vi "Lectura Silicon 6 bytes.vi"() -> ()   [LabVIEW 2013]
uses:
  <vilib>/Instr/_visa.llb/VISA Configure Serial Port (Instr).vi
  <vilib>/Instr/_visa.llb/VISA Serial Break (Instr).vi
panel:
  out "array 2":string[](array[string])
  out "read buffer 2":string
  out "Waveform Graph 2":waveform(i32)(graph)
  in  "Reiniciar":bool
  out "mps":dbl
  out "Array 3":string[](array[string])
  out "Array 2":timestamp[](array[timestamp])
  out "unsigned byte array":u8[](array[numeric])
  out "x != y?":bool
  in  "Array":bool[](array[boolean])=[FALSE, FALSE, FALSE, FALSE, FALSE, FALSE, FALSE, TRUE]
  out "Waveform Graph":waveform(i32)(graph)
  out "Boolean array":bool[][](array[boolean])
  out "array":string[](array[string])
  in  "stop":bool
  out "read buffer":string
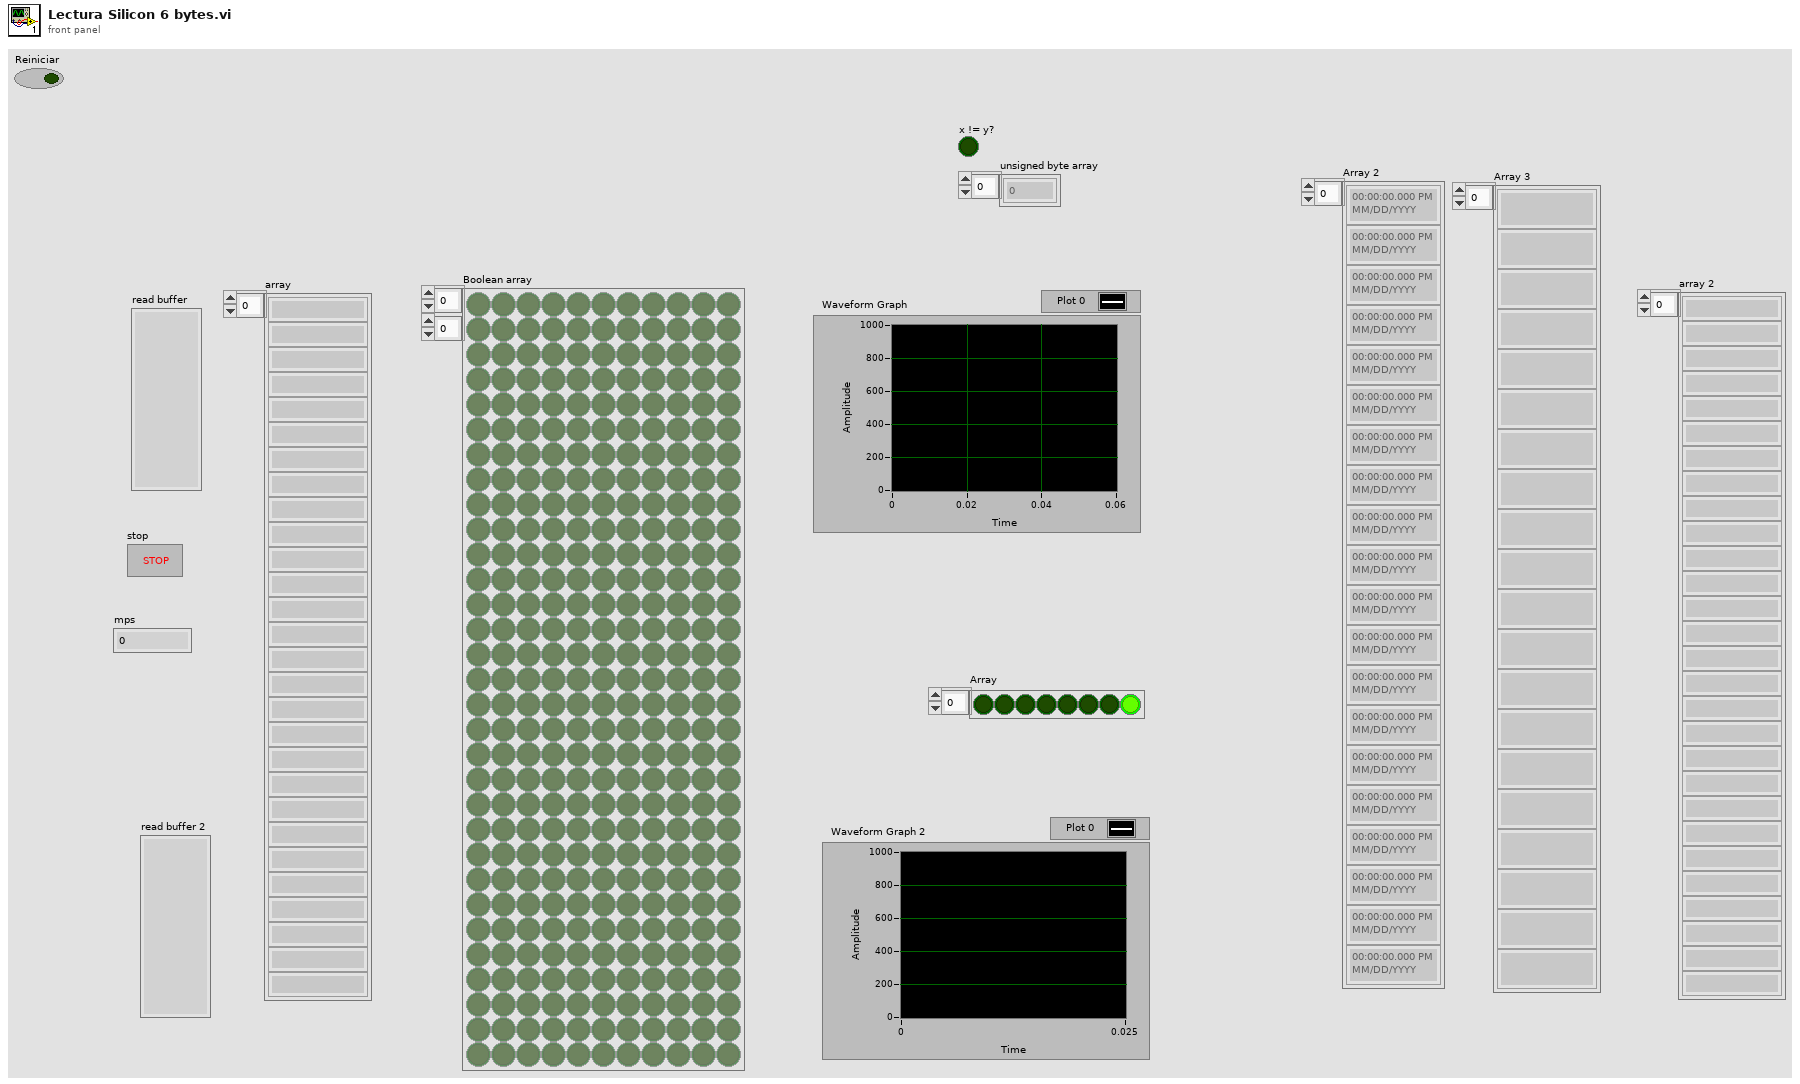
[diagram p1: front panel]
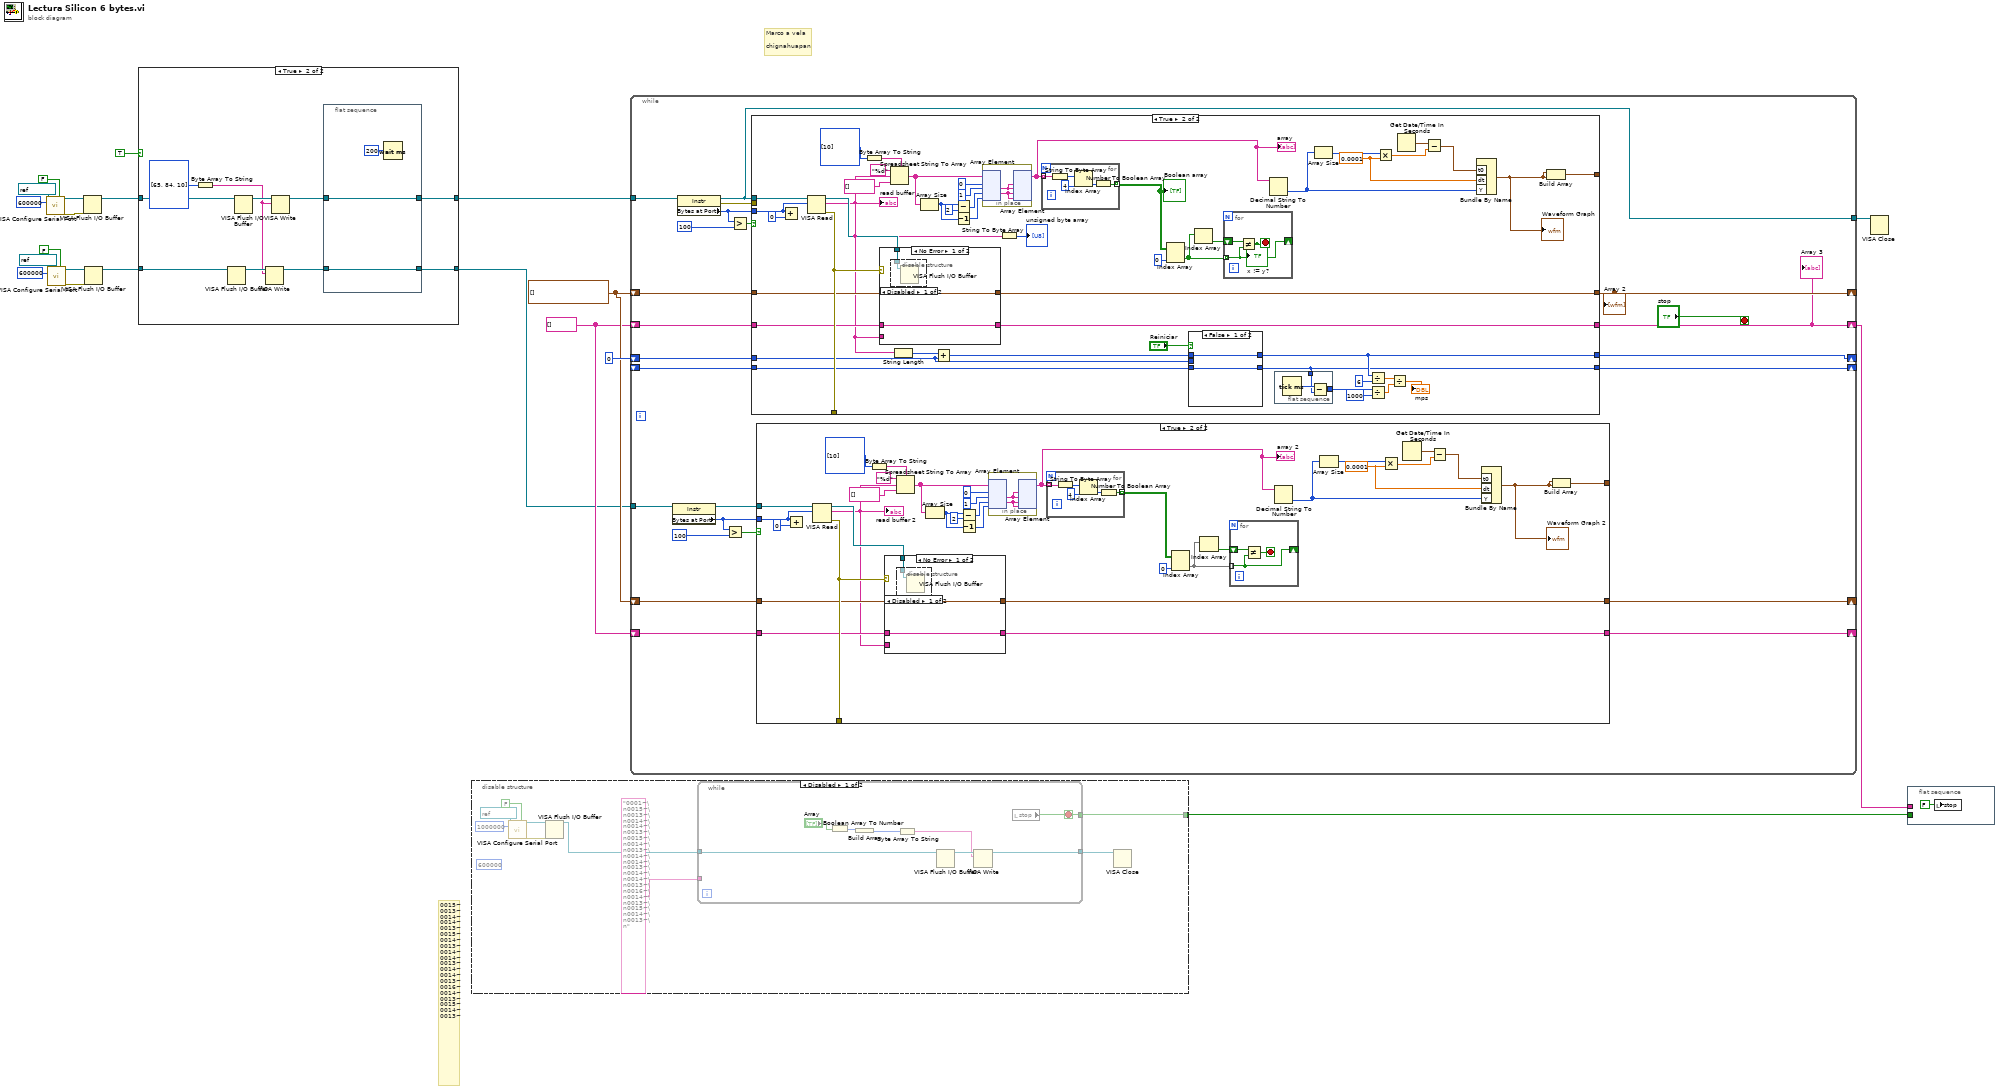
[diagram p0: block diagram]
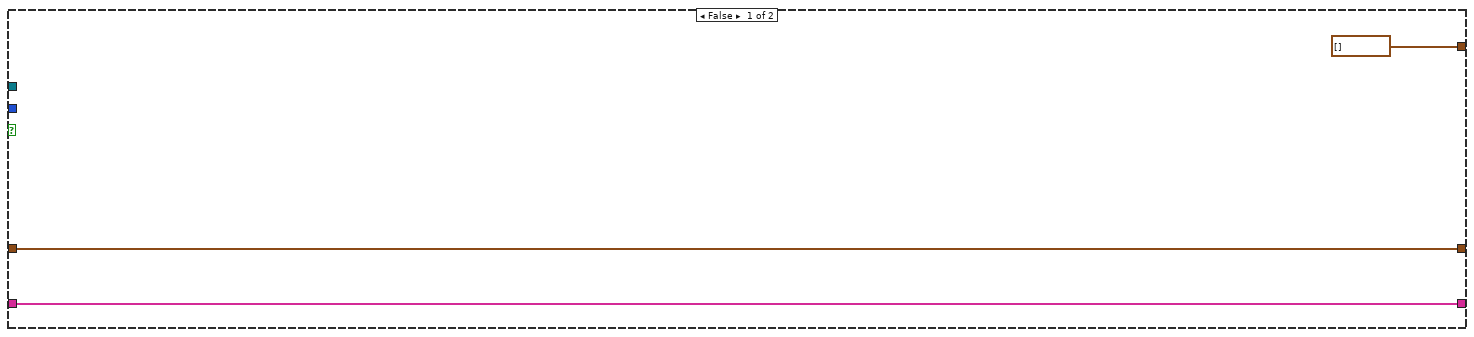
[diagram p4: hidden frame]
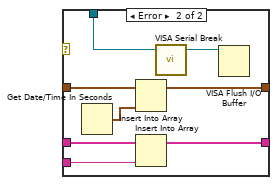
[diagram p6: hidden frame]
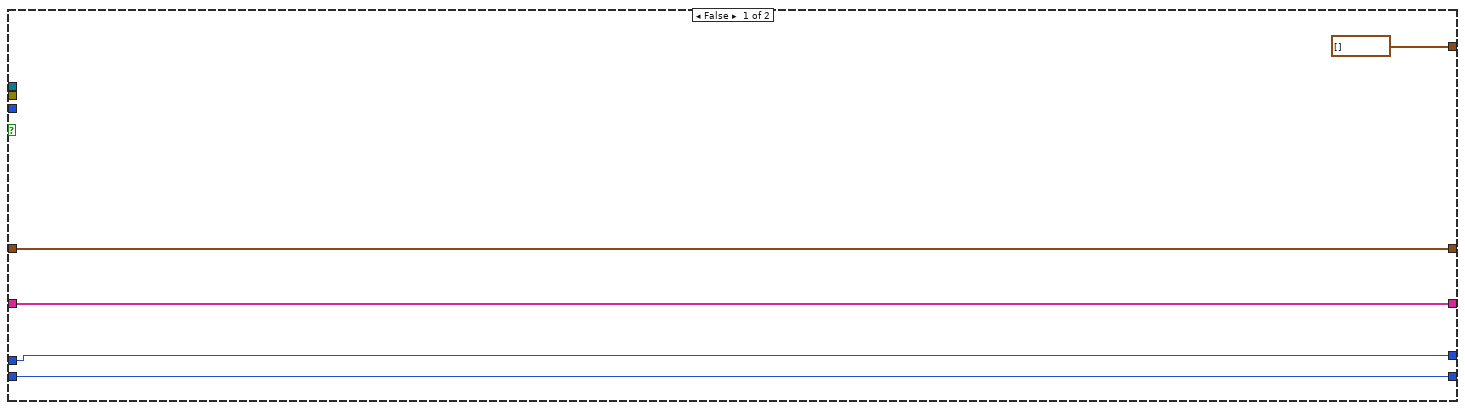
[diagram p7: hidden frame]
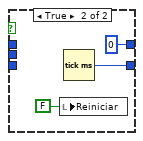
[diagram p8: hidden frame]
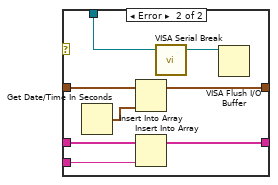
[diagram p10: hidden frame]
diagram:
  w8 = string[] []
  w9 = timestamp[] []
  # "Marco a vela\n\nchignahuapan"
  # "0015~\n0013~\n0014~\n0014~\n0013~\n0015~\n0014~\n0013~\n0014~\n0014~\n0013~\n0014~\n0014~\n0013~\n0016~\n0014~\n0013~\n0015~\n0014~\n0013~"
  n1 = call-poly "VISA Configure Serial Port"("VISA resource name"=refnum<visa-resource-name> "COM4", "Enable Termination\nChar (T)"=FALSE ("Enable Termination\nChar (T)"), "baud rate (9600)"=u32 600000) -> ("VISA resource name out"=w19:refnum<visa-resource-name>, "error out"=w18:errorcluster)  [unwired: 11 in]
  n2 = call-poly "VISA Configure Serial Port"("VISA resource name"=refnum<visa-resource-name> "COM5", "Enable Termination\nChar (T)"=FALSE ("Enable Termination\nChar (T)"), "baud rate (9600)"=u32 600000) -> ("VISA resource name out"=w5:refnum<visa-resource-name>, "error out"=w6:errorcluster)  [unwired: 11 in]
  n3 = VISA Flush I/O Buffer(VISA resource name=w19, error in (no error)=w18) -> (VISA resource name out=w12:refnum<visa-resource-name>)  [unwired: 1 in, 1 out]
  n4 = VISA Flush I/O Buffer(VISA resource name=w5, error in (no error)=w6) -> (VISA resource name out=w2:refnum<visa-resource-name>)  [unwired: 1 in, 1 out]
  n5 = case shown="True" TRUE {
    tunnel: w12 -> [w23 w32]
    tunnel: [w23 w29] -> w11
    tunnel: w2 -> [w22 w27]
    tunnel: [w22 w24] -> w1
    frame False {
    }
    frame True {
      n6 = Byte Array To String(unsigned byte array=u8[] [65, 84, 10]) -> (string=w26:string)
      n7 = VISA Flush I/O Buffer(VISA resource name=w27) -> (VISA resource name out=w28:refnum<visa-resource-name>)  [unwired: 2 in, 1 out]
      n8 = VISA Flush I/O Buffer(VISA resource name=w32) -> (VISA resource name out=w33:refnum<visa-resource-name>)  [unwired: 2 in, 1 out]
      n9 = VISA Write(VISA resource name=w28, write buffer=w26) -> (VISA resource name out=w25:refnum<visa-resource-name>)  [unwired: 1 in, 2 out]
      n10 = VISA Write(VISA resource name=w33, write buffer=w26) -> (VISA resource name out=w30:refnum<visa-resource-name>)  [unwired: 1 in, 2 out]
      n11 = flat-sequence {
        tunnel: w30 -> [w36]
        tunnel: [w36] -> w29
        tunnel: w25 -> [w34]
        tunnel: [w34] -> w24
        frame #0 {
          n12 = Wait (ms)(milliseconds to wait=u32 200) -> ()  [unwired: 1 out]
        }
      }
    }
  }
  n13 = disable-structure shown="Disabled" {
    disable-tunnel: [w40 _] -> w14
    frame Disabled {
      (unwired) u32 600000 ("baud rate (9600)")
      n14 = call-poly "VISA Configure Serial Port"("VISA resource name"=refnum<visa-resource-name> "COM5", "Enable Termination\nChar (T)"=FALSE ("Enable Termination\nChar (T)"), "baud rate (9600)"=u32 1000000) -> ("VISA resource name out"=w43:refnum<visa-resource-name>, "error out"=w44:errorcluster)  [unwired: 11 in]
      n15 = VISA Flush I/O Buffer(VISA resource name=w43, error in (no error)=w44) -> (VISA resource name out=w41:refnum<visa-resource-name>)  [unwired: 1 in, 1 out]
      n16 = while {
        tunnel: w41 -> [w49]
        tunnel: [w48] -> w40
        tunnel: "0001~\n0015~\n0013~\n0014~\n0014~\n0013~\n0015~\n0014~\n0013~\n0014~\n0014~\n0013~\n0014~\n0014~\n0013~\n0016~\n0014~\n0013~\n0015~\n0014~\n0013~\n" ("read buffer") -> [_]
        tunnel: [w47] -> w38
        stop <- w48 stop-if-true
        n17 = Boolean Array To Number(Boolean array="Array") -> (number=w52:u8)
        n18 = Build Array(w52) -> (w53:u8[])
        n19 = Byte Array To String(unsigned byte array=w53) -> (string=w46:string)
        n20 = VISA Flush I/O Buffer(VISA resource name=w49) -> (VISA resource name out=w50:refnum<visa-resource-name>)  [unwired: 2 in, 1 out]
        n21 = VISA Write(VISA resource name=w50, write buffer=w46) -> (VISA resource name out=w47:refnum<visa-resource-name>)  [unwired: 1 in, 2 out]
        n22 = local read "stop"() -> (w48:bool)
      }
      n23 = VISA Close(VISA resource name=w38) -> ()  [unwired: 1 in, 1 out]
    }
    frame Enabled {
    }
  }
  n24 = while {
    tunnel: w11 -> [w73]
    tunnel: [w72] -> w16
    shift-right: [w70] -> _
    shift-left: w9 -> [w71]
    shift-right: [w68] -> w15
    shift-left: w8 -> [w69]
    shift-right: [w65] -> _
    shift-left: u32 0 ("length") -> [w66]
    shift-right: [w64] -> _
    shift-left: _ -> [w63]
    shift-right: [w60] -> _
    shift-left: w9 -> [w62]
    shift-right: [w59] -> _
    shift-left: w8 -> [w61]
    tunnel: w1 -> [w56]
    stop <- "stop" stop-if-true
    n25 = property class="Instr"(reference=w56) -> (reference out=w55:refnum<visa-resource-name>, "Bytes at Port"=w54:u32)  [unwired: 1 in, 1 out]
    n26 = property class="Instr"(reference=w73) -> (reference out=w72:refnum<visa-resource-name>, error out=w76:errorcluster, "Bytes at Port"=w77:u32)  [unwired: 1 in]
    n27 = Greater?(x=w54, y=u32 100) -> (0:w57:bool)
    n28 = Greater?(x=w77, y=u32 100) -> (0:w67:bool)
    n29 = case shown="True" w67 {
      tunnel: w72 -> [_ w164]
      tunnel: w77 -> [_ w156]
      tunnel: [waveform(dbl)[] [] w180] -> _
      tunnel: w76 -> [_ _]
      tunnel: [_ w163] -> _
      tunnel: w71 -> [w140 w161]
      tunnel: [w140 w160] -> w70
      tunnel: w69 -> [w139 w159]
      tunnel: [w139 w158] -> w68
      tunnel: w66 -> [w138 w145]
      tunnel: [w138 w144] -> w65
      tunnel: [w137 w142] -> w64
      tunnel: w63 -> [w137 w151]
      frame False {
      }
      frame True {
        w184 = 0.0001 ("dt")
        n30 = Add(x=w156, y=u32 0) -> ()  [unwired: 1 out]
        n31 = VISA Read(VISA resource name=w164, byte count=w156) -> (VISA resource name out=w162:refnum<visa-resource-name>, read buffer=w155:string, error out=w163:errorcluster)  [unwired: 1 in, 1 out]
        "read buffer" <- w155
        n32 = Byte Array To String(unsigned byte array=u8[] [10]) -> (string=w187:string)
        n33 = case shown="No Error" w163 {
          tunnel: w162 -> [w198 w206]
          tunnel: w161 -> [w200 w209]
          tunnel: [w200 w208] -> w160
          tunnel: w159 -> [w199 w204]
          tunnel: w155 -> [_ w203]
          tunnel: [w199 w202] -> w158
          frame No Error {
            n34 = disable-structure shown="Disabled" {
              disable-tunnel: w198 -> [w201 _]
              frame Disabled {
                n35 = VISA Flush I/O Buffer(VISA resource name=w201) -> ()  [unwired: 2 in, 2 out]
              }
              frame Enabled {
              }
            }
          }
          frame Error {
            n36 = Get Date/Time In Seconds() -> (seconds since 1Jan1904=w207:timestamp)
            n37 = Insert Into Array(array=w209, new element=w207) -> (w208:timestamp[])  [unwired: 1 in]
            n38 = Insert Into Array(array=w204, new element=w203) -> (w202:string[])  [unwired: 1 in]
            n39 = call-poly <vilib>:"VISA Serial Break.vi"("VISA resource name"=w206) -> ("VISA resource name out"=w205:refnum<visa-resource-name>)  [unwired: 3 in, 1 out]
            n40 = VISA Flush I/O Buffer(VISA resource name=w205) -> ()  [unwired: 2 in, 2 out]
          }
        }
        n41 = Spreadsheet String To Array(delimiter (Tab)=w187, format string="%d", spreadsheet string=w155, array type (2D Dbl)=string[] []) -> (array=w170:string[])
        n42 = String Length(string=w155) -> (length=w154:i32)
        n43 = Array Size(array=w170) -> (size(s)=w173:i32)
        n44 = Add(x=w154, y=w145) -> (x+y=w152:u32)
        n45 = Subtract(x=w173, y=2) -> (x-y=w177:i32)
        n46 = Decrement(x=w173) -> (x-1=w172:i32)
        n47 = in-place {
          n48 = in-place-array #1(w170, 0, 1, w177, w172) -> (w214:string, w213:string)  [unwired: 2 out]
          n49 = in-place-array #1(w214, w214, w213, w213) -> (w171:string[])  [unwired: 4 out]
        }
        "array" <- w171
        n50 = String To Byte Array(string=w155) -> (unsigned byte array=→"unsigned byte array":u8[])
        n51 = for {
          tunnel: w171 -> [w216] mode=indexing
          tunnel: [w217] -> w169 mode=indexing
          n52 = String To Byte Array(string=w216) -> (unsigned byte array=w219:u8[])
          n53 = Index Array(array=w219, index=4) -> (element=w218:u8)
          n54 = Number To Boolean Array(number=w218) -> (Boolean array=w217:bool[])
        }
        "Boolean array" <- w169
        n55 = Index Array(array=w169, index (col)=0 ("disabled index (col)")) -> (element=w167:bool[])  [unwired: 1 in]
        n56 = case shown="False" "Reiniciar" {
          tunnel: w152 -> [w194 _]
          tunnel: [w194 u32 0] -> w144
          tunnel: [w193 w196] -> w142
          tunnel: w151 -> [w193 _]
          tunnel: w145 -> [_ _]
          frame False {
          }
          frame True {
            n57 = local write "Reiniciar"(FALSE ("Reiniciar")) -> ()
            n58 = Tick Count (ms)() -> (millisecond timer value=w196:u32)
          }
        }
        n59 = Index Array(array=w167) -> (element=w166:bool)  [unwired: 1 in]
        n60 = for {
          tunnel: w167 -> [w211] mode=indexing
          shift-right: [w211] -> _
          shift-left: w166 -> [w212]
          stop <- w210 stop-if-true
          n61 = Not Equal?(x=w212, y=w211) -> (x != y?=w210:bool)
          "x != y?" <- w210
        }
        n62 = Decimal String To Number(string=w171) -> (number=w179:i32[])  [unwired: 2 in, 1 out]
        n63 = flat-sequence {
          tunnel: [w192] -> w147
          tunnel: w142 -> [w190]
          frame #0 {
            n64 = Tick Count (ms)() -> (millisecond timer value=w191:u32)
            n65 = Subtract(x=w191, y=w190) -> (x-y=w192:u32)
          }
        }
        n66 = Array Size(array=w179) -> (size(s)=w183:i32)
        n67 = Divide(x=w144, y=6) -> (x/y=w143:dbl)
        n68 = Divide(x=w147, y=u32 1000) -> (x/y=w149:dbl)
        n69 = Multiply(x=w183, y=w184) -> (x*y=w182:dbl)
        n70 = Divide(x=w143, y=w149) -> (x/y=→"mps":dbl)
        n71 = Get Date/Time In Seconds() -> (seconds since 1Jan1904=w185:timestamp)
        n72 = Subtract(x=w185, y=w182) -> (x-y=w181:timestamp)
        n73 = Bundle By Name("t0"=w181, "dt"=w184, "Y"=w179) -> (w178:waveform(i32))  [unwired: 1 in]
        "Waveform Graph" <- w178
        n74 = Build Array(w178, w178) -> (w180:waveform(i32)[])
      }
    }
    "Array 2" <- w70
    "Array 3" <- w68
    n75 = case shown="True" w57 {
      tunnel: w55 -> [_ w91]
      tunnel: w54 -> [_ w83]
      tunnel: [waveform(dbl)[] [] w105] -> _
      tunnel: [_ w90] -> _
      tunnel: w62 -> [w79 w88]
      tunnel: [w79 w87] -> w60
      tunnel: w61 -> [w78 w86]
      tunnel: [w78 w85] -> w59
      frame False {
      }
      frame True {
        w109 = 0.0001 ("dt")
        n76 = Add(x=w83, y=u32 0) -> ()  [unwired: 1 out]
        n77 = VISA Read(VISA resource name=w91, byte count=w83) -> (VISA resource name out=w89:refnum<visa-resource-name>, read buffer=w82:string, error out=w90:errorcluster)  [unwired: 1 in, 1 out]
        "read buffer 2" <- w82
        n78 = Byte Array To String(unsigned byte array=u8[] [10]) -> (string=w112:string)
        n79 = case shown="No Error" w90 {
          tunnel: w89 -> [w115 w123]
          tunnel: w88 -> [w117 w126]
          tunnel: [w117 w125] -> w87
          tunnel: w86 -> [w116 w121]
          tunnel: w82 -> [_ w120]
          tunnel: [w116 w119] -> w85
          frame No Error {
            n80 = disable-structure shown="Disabled" {
              disable-tunnel: w115 -> [w118 _]
              frame Disabled {
                n81 = VISA Flush I/O Buffer(VISA resource name=w118) -> ()  [unwired: 2 in, 2 out]
              }
              frame Enabled {
              }
            }
          }
          frame Error {
            n82 = Get Date/Time In Seconds() -> (seconds since 1Jan1904=w124:timestamp)
            n83 = Insert Into Array(array=w126, new element=w124) -> (w125:timestamp[])  [unwired: 1 in]
            n84 = Insert Into Array(array=w121, new element=w120) -> (w119:string[])  [unwired: 1 in]
            n85 = call-poly <vilib>:"VISA Serial Break.vi"("VISA resource name"=w123) -> ("VISA resource name out"=w122:refnum<visa-resource-name>)  [unwired: 3 in, 1 out]
            n86 = VISA Flush I/O Buffer(VISA resource name=w122) -> ()  [unwired: 2 in, 2 out]
          }
        }
        n87 = Spreadsheet String To Array(delimiter (Tab)=w112, format string="%d", spreadsheet string=w82, array type (2D Dbl)=string[] []) -> (array=w96:string[])
        n88 = Array Size(array=w96) -> (size(s)=w98:i32)
        n89 = Subtract(x=w98, y=2) -> (x-y=w102:i32)
        n90 = Decrement(x=w98) -> (x-1=w97:i32)
        n91 = in-place {
          n92 = in-place-array #2(w96, 0, 1, w102, w97) -> (w131:string, w130:string)  [unwired: 2 out]
          n93 = in-place-array #2(w131, w131, w130, w130) -> (w81:string[])  [unwired: 4 out]
        }
        "array 2" <- w81
        n94 = for {
          tunnel: w81 -> [w133] mode=indexing
          tunnel: [w134] -> w95 mode=indexing
          n95 = String To Byte Array(string=w133) -> (unsigned byte array=w136:u8[])
          n96 = Index Array(array=w136, index=4) -> (element=w135:u8)
          n97 = Number To Boolean Array(number=w135) -> (Boolean array=w134:bool[])
        }
        n98 = Index Array(array=w95, index (col)=0 ("disabled index (col)")) -> (element=w93:bool[])  [unwired: 1 in]
        n99 = Index Array(array=w93) -> (element=w92:bool)  [unwired: 1 in]
        n100 = for {
          tunnel: w93 -> [w128] mode=indexing
          shift-right: [w128] -> _
          shift-left: w92 -> [w129]
          stop <- w127 stop-if-true
          n101 = Not Equal?(x=w129, y=w128) -> (x != y?=w127:bool)
        }
        n102 = Decimal String To Number(string=w81) -> (number=w104:i32[])  [unwired: 2 in, 1 out]
        n103 = Array Size(array=w104) -> (size(s)=w108:i32)
        n104 = Multiply(x=w108, y=w109) -> (x*y=w107:dbl)
        n105 = Get Date/Time In Seconds() -> (seconds since 1Jan1904=w110:timestamp)
        n106 = Subtract(x=w110, y=w107) -> (x-y=w106:timestamp)
        n107 = Bundle By Name("t0"=w106, "dt"=w109, "Y"=w104) -> (w103:waveform(i32))  [unwired: 1 in]
        "Waveform Graph 2" <- w103
        n108 = Build Array(w103, w103) -> (w105:waveform(i32)[])
      }
    }
  }
  n109 = VISA Close(VISA resource name=w16) -> ()  [unwired: 1 in, 1 out]
  n110 = flat-sequence {
    tunnel: w15 -> [_]
    tunnel: w14 -> [_]
    frame #0 {
      n111 = local write "stop"(FALSE ("stop")) -> ()
    }
  }
